vi "Set Main Settings.vi"(8 "error in":errorcluster, 10 "settings":T2, 11 "scan engine custom device ref in":T1 format="%.0x") -> (0 "error out":errorcluster, 3 "scan engine custom device ref out":T1 format="%.0x")   [LabVIEW 2019, in "SEECD System Explorer.lvlib"]
uses:
  SEECD System Explorer.lvlib
  Shared/Type Defs/Main Settings.ctl
  <vilib>/NI VeriStand/Custom Device API/Custom Device Item Ref.ctl
  Scripting/Scan Engine Scripting.lvlib
  Shared/SEECD Shared.lvlib
  <vilib>/NI VeriStand/Custom Device API/Custom Device API.lvlib
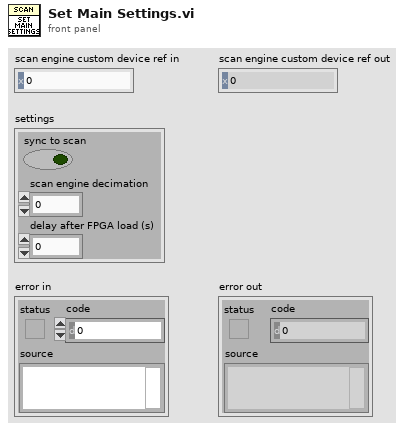
[diagram p1: front panel]
types:
  T1 = typedef "Custom Device API.lvlib/Custom Device Item Ref.ctl" = u64
  T2 = typedef "SEECD Shared.lvlib/Main Settings.ctl" = cluster{"sync to scan":bool, "scan engine decimation":u16, "delay after FPGA load (s)":u16}
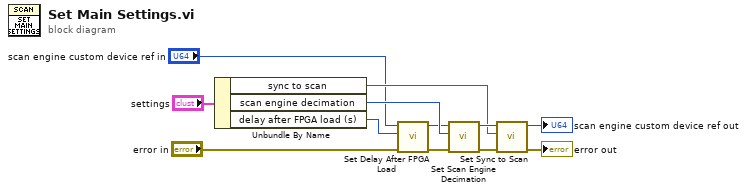
[diagram p0: block diagram]
diagram:
  n1 = Unbundle By Name("settings") -> ("sync to scan"=w10:bool, "scan engine decimation"=w9:u16, "delay after FPGA load (s)"=w1:u16)
  n2 = call "Set Delay After FPGA Load.vi"("error in"="error in", "delay after FPGA load (s)"=w1, "scan engine custom device ref in"="scan engine custom device ref in") -> ("error out"=w4:errorcluster, "scan engine custom device ref out"=w5:T1)  [unwired: 7 in]
  n3 = call "Set Scan Engine Decimation.vi"("error in"=w4, "scan engine decimation"=w9, "scan engine custom device ref in"=w5) -> ("error out"=w11:errorcluster, "scan engine custom device ref out"=w12:T1)  [unwired: 7 in]
  n4 = call "Set Sync to Scan.vi"("error in"=w11, "sync to scan"=w10, "scan engine custom device ref in"=w12) -> ("error out"=→"error out":errorcluster, "scan engine custom device ref out"=→"scan engine custom device ref out":T1)  [unwired: 7 in]
